vi "rotate phase angle of graph.vi"() -> ()   [LabVIEW 2012]
doc: "Rotates the phase of XY data from a Lockin Amplifier.\nWill average multiple input files.\nOnly use multiple files with the same scan parameters."
uses:
  <vilib>/Analysis/baseanly.llb/Mean (DBL).vi
  <vilib>/Utility/file.llb/Write To Spreadsheet File (DBL).vi
  <vilib>/Analysis/NI_AALBase.lvlib
panel:
  in  "Theta":dbl(knob) scale=0.0..360.0
  out "StdDev of Y":sgl
  out "#pages":i32
  out "#columns":i32
  out "#rows":i32
  in  "Put each data file you want to \naverage into a separate array element":string[](array[string])
  in  "Read in from array":bool
  out "array of new data":dbl[][](array[numeric])
  in  "Output to .xls file":bool
  in  "stop":bool
  out "Rotated Graph":T1(graph) caption="cpsgraph"
  in  "Original Graph":T2(graph) caption="cpsgraph"
  # "(pops up dialog box for name)"
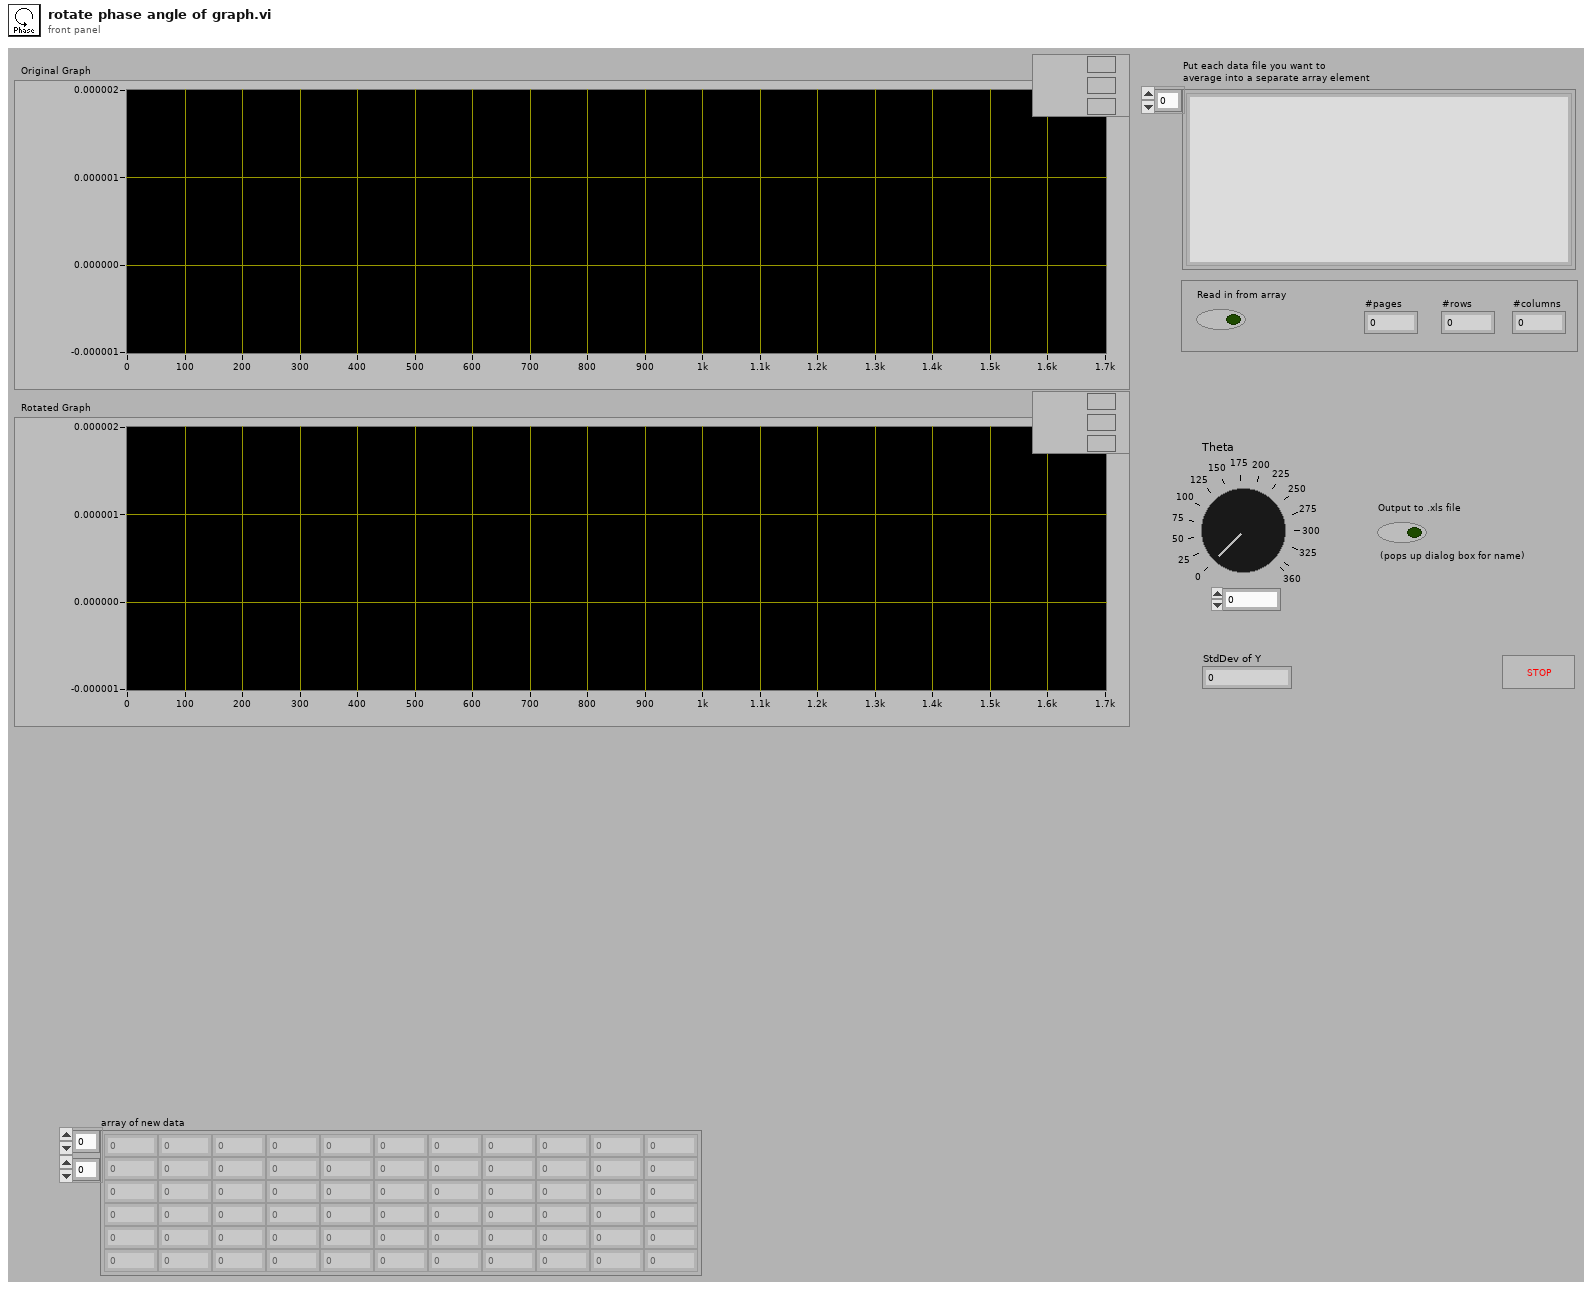
[diagram p1: front panel]
types:
  T1 = cluster{"point array":cluster{"x":dbl, "y":dbl}[]}[]
  T2 = typedef "Scan Driver.lvclass/Scan Graph.ctl" = cluster{"point array":cluster{"x":dbl, "y":dbl}[]}[]
  T3 = cluster{"point array":cluster{"x":dbl, "y":dbl}[]}
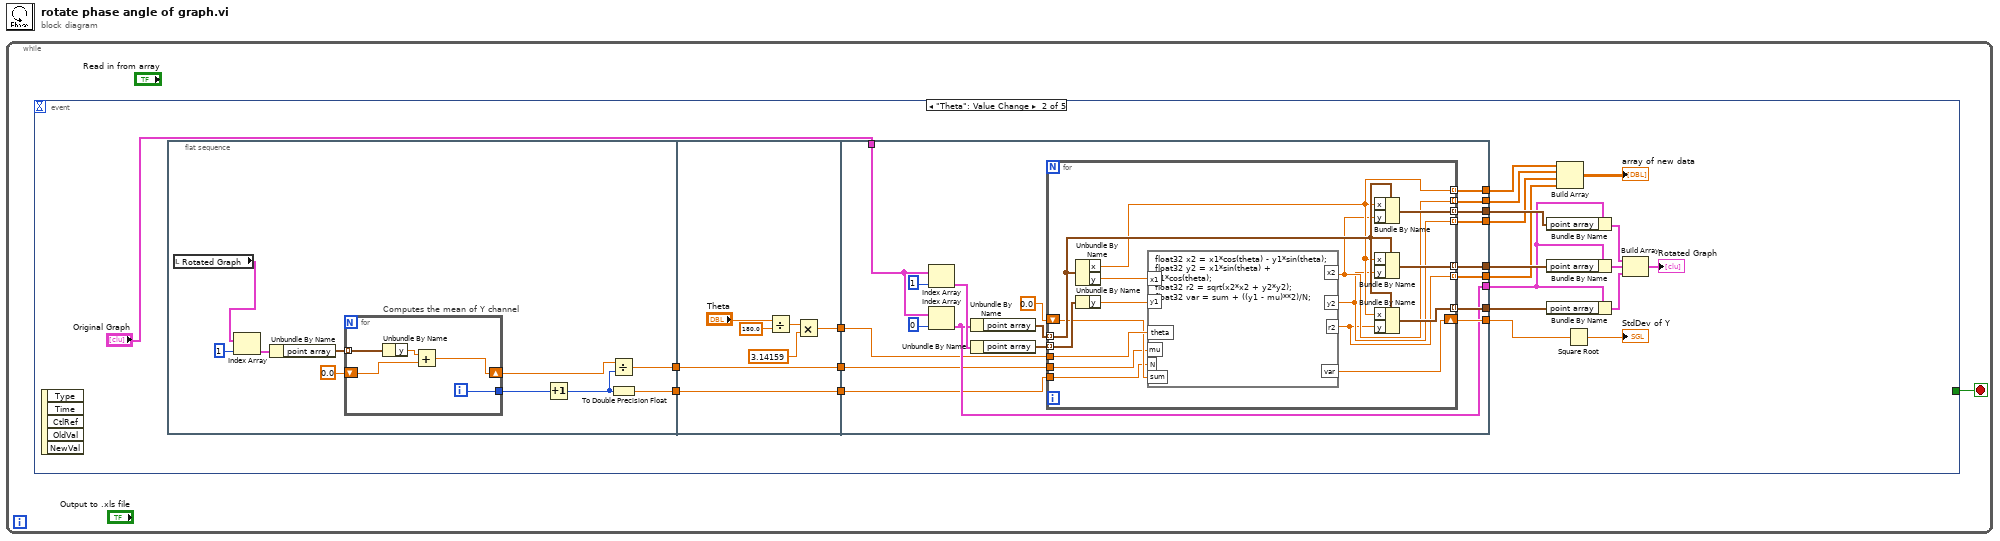
[diagram p0: block diagram]
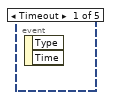
[diagram p2: hidden frame]
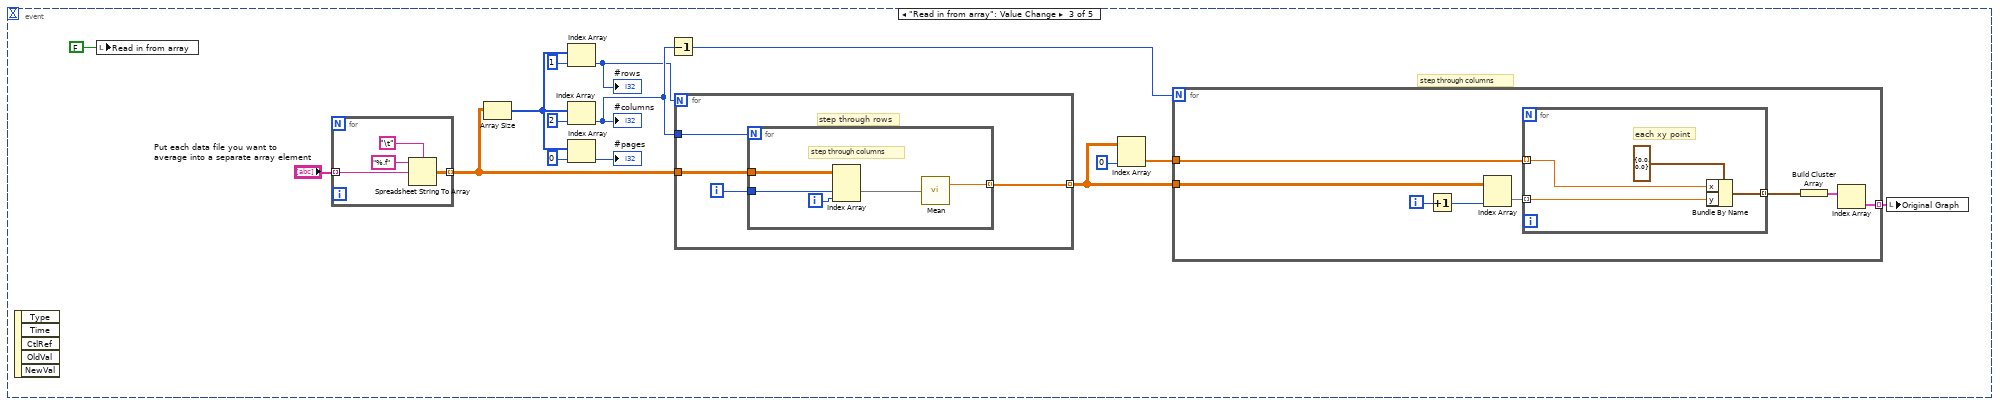
[diagram p3: hidden frame]
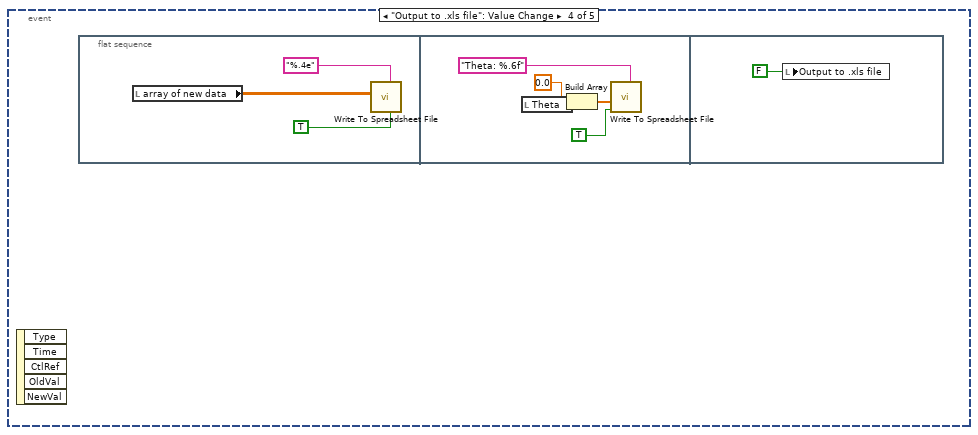
[diagram p4: hidden frame]
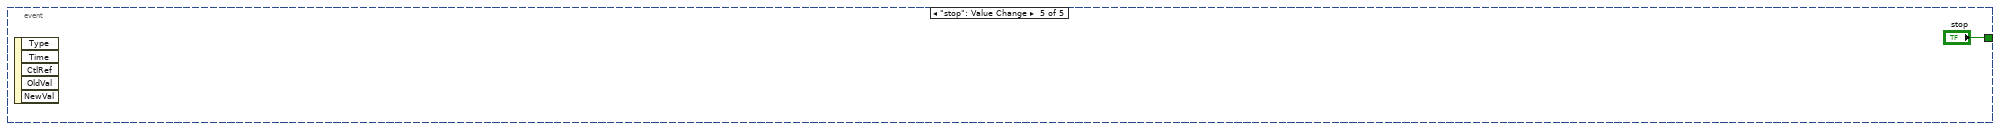
[diagram p5: hidden frame]
diagram:
  n1 = while {
    stop <- w1 stop-if-true
    n2 = event shown="[1] \"Theta\": Value Change" {
      selector: _ -> [_ _ _ _ _]
      dyn-events: _ -> [_ _ _ _ _]
      timeout: _ -> [_ _ _ _ _]
      tunnel: [_ _ _ _ "stop"] -> w1
      event Timeout {
        n3 = event-data() -> ()  [unwired: 1 in, 2 out]
      }
      event "Theta": Value Change {
        n4 = event-data() -> ()  [unwired: 1 in, 5 out]
        n5 = flat-sequence {
          tunnel: [w25] -> w6
          tunnel: [w24] -> w4
          tunnel: w6 -> [w39]
          tunnel: [w40] -> w5
          tunnel: w4 -> [w40]
          tunnel: [w39] -> w3
          tunnel: [w38] -> w2
          tunnel: [w63] -> w18
          tunnel: [w62] -> w17
          tunnel: [w61] -> w16
          tunnel: [w60] -> w15
          tunnel: [w59] -> w14
          tunnel: [w58] -> w13
          tunnel: [w57] -> w12
          tunnel: [w56] -> w10
          tunnel: "Original Graph" -> [w50]
          tunnel: [w49] -> w8
          tunnel: w5 -> [w48]
          tunnel: w3 -> [w47]
          tunnel: w2 -> [w46]
          frame #0 {
            n6 = local read "Rotated Graph"() -> (w23:T1)
            n7 = Index Array(array=w23, index=1) -> (element=w26:T3)
            n8 = Unbundle By Name(w26) -> ("point array"=w27:cluster{"x":dbl, "y":dbl}[])
            n9 = for "Computes the mean of Y channel" {
              tunnel: w27 -> [w34] mode=indexing
              shift-right: [w36] -> w30
              shift-left: 0.0 -> [w37]
              tunnel: [w35] -> w29
              i -> [w35]
              n10 = Unbundle By Name(w34) -> ("y"=w33:dbl)
              n11 = Add(x=w33, y=w37) -> (x+y=w36:dbl)
            }
            n12 = Increment(x=w29) -> (x+1=w31:i32)
            n13 = Divide(x=w30, y=w31) -> (x/y=w25:dbl)
            n14 = To Double Precision Float(number=w31) -> (double precision float=w24:dbl)
          }
          frame #1 {
            n15 = Divide(x="Theta", y=180.0) -> (x/y=w42:dbl)
            n16 = Multiply(x=w42, y=3.14159) -> (x*y=w38:dbl)
          }
          frame #2 {
            n17 = Index Array(array=w50, index=1) -> (element=w53:T3)
            n18 = Index Array(array=w50, index=0) -> (element=w49:T3)
            n19 = Unbundle By Name(w49) -> ("point array"=w52:cluster{"x":dbl, "y":dbl}[])
            n20 = Unbundle By Name(w53) -> ("point array"=w51:cluster{"x":dbl, "y":dbl}[])
            n21 = for {
              tunnel: w52 -> [w78] mode=indexing
              tunnel: w51 -> [w79] mode=indexing
              tunnel: w46 -> [w71]
              tunnel: [w77] -> w61 mode=indexing
              tunnel: [w76] -> w62 mode=indexing
              tunnel: [w75] -> w63 mode=indexing
              tunnel: [w74] -> w60 mode=indexing
              tunnel: [w70] -> w59 mode=indexing
              tunnel: [w69] -> w58 mode=indexing
              tunnel: [w68] -> w57 mode=indexing
              shift-right: [w67] -> w56
              shift-left: sgl 0.0 -> [w66]
              tunnel: w48 -> [w65]
              tunnel: w47 -> [w64]
              n22 = Unbundle By Name(w78) -> ("x"=w74:dbl, "y"=w73:dbl)
              n23 = Unbundle By Name(w79) -> ("y"=w72:dbl)
              n24 = formula code="float32 x2 = x1*cos(theta) - y1*sin(theta);\nfloat32 y2 = x1*sin(theta) + y1*cos(theta);\nfloat32 r2 = sqrt(x2*x2 + y2*y2);\nfloat32 var = sum + ((y1 - mu)**2)/N;"("x1"=w73, "y1"=w72, "theta"=w71, "mu"=w64, "N"=w65, "sum"=w66) -> ("x2"=w70:sgl, "y2"=w69:sgl, "r2"=w68:sgl, "var"=w67:sgl)
              n25 = Bundle By Name(cluster=w78, "x"=w74, "y"=w70) -> (w77:cluster{"x":dbl, "y":dbl})
              n26 = Bundle By Name(cluster=w78, "x"=w74, "y"=w69) -> (w76:cluster{"x":dbl, "y":dbl})
              n27 = Bundle By Name(cluster=w78, "x"=w74, "y"=w68) -> (w75:cluster{"x":dbl, "y":dbl})
            }
          }
        }
        n28 = Bundle By Name(cluster=w8, "point array"=w16) -> (w19:T3)
        n29 = Bundle By Name(cluster=w8, "point array"=w17) -> (w20:T3)
        n30 = Bundle By Name(cluster=w8, "point array"=w18) -> (w21:T3)
        n31 = Build Array(w15, w14, w13, w12) -> (→"array of new data":dbl[][])
        n32 = Square Root(x=w10) -> (sqrt(x)=→"StdDev of Y":sgl)
        n33 = Build Array(w19, w20, w21) -> (→"Rotated Graph":T1)
      }
      event "Read in from array": Value Change {
        # "step through columns"
        n34 = event-data() -> ()  [unwired: 1 in, 5 out]
        n35 = local write "Read in from array"(FALSE ("Read in from array")) -> ()
        n36 = for {
          tunnel: "Put each data file you want to \naverage into a separate array element" -> [w119] mode=indexing
          tunnel: [w118] -> w81 mode=indexing
          n37 = Spreadsheet String To Array(delimiter (Tab)="\t", format string="%.f", spreadsheet string=w119) -> (array=w118:dbl[][])  [unwired: 1 in]
        }
        n38 = Array Size(array=w81) -> (size(s)=w91:i32[])
        n39 = Index Array(array=w91, index=1) -> (element=w80:i32)
        "#rows" <- w80
        n40 = Index Array(array=w91, index=2) -> (element=w87:i32)
        "#columns" <- w87
        n41 = Index Array(array=w91, index=0) -> (element=→"#pages":i32)
        n42 = Decrement(x=w87) -> (x-1=w86:i32)
        n43 = for {
          N: w80 -> [_]
          tunnel: w81 -> [w110]
          tunnel: [w109] -> w83 mode=indexing
          tunnel: w87 -> [w108]
          i -> [w107]
          # "step through rows"
          n44 = for {
            N: w108 -> [_]
            tunnel: w110 -> [w114]
            tunnel: [w115] -> w109 mode=indexing
            tunnel: w107 -> [w113]
            i -> [w112]
            # "step through columns"
            n45 = Index Array(array=w114, index (dim 1)=w113, index (dim 2)=w112) -> (element=w111:dbl[])  [unwired: 1 in]
            n46 = call-poly <vilib>:"Mean.vi"("X"=w111) -> ("mean"=w115:dbl)  [unwired: 1 out]
          }
        }
        n47 = Index Array(array=w83, index (col)=0 ("disabled index (col)")) -> (element=w82:dbl[])  [unwired: 1 in]
        n48 = for {
          N: w86 -> [_]
          tunnel: w83 -> [w99]
          tunnel: [w95] -> w85 mode=indexing
          tunnel: w82 -> [w98]
          i -> [w100]
          n49 = Increment(x=w100) -> (x+1=w102:i32)
          n50 = Index Array(array=w99, index (col)=w102) -> (element=w101:dbl[])  [unwired: 1 in]
          n51 = for {
            tunnel: w98 -> [w106] mode=indexing
            tunnel: w101 -> [w105] mode=indexing
            tunnel: [w104] -> w97 mode=indexing
            # "each xy point"
            n52 = Bundle By Name(cluster=cluster{"x":dbl, "y":dbl} {"x"=0.0, "y"=0.0} ("element"), "x"=w106, "y"=w105) -> (w104:cluster{"x":dbl, "y":dbl})
          }
          n53 = Build Cluster Array(w97) -> (w96:cluster{cluster{"x":dbl, "y":dbl}[]}[])
          n54 = Index Array(array=w96) -> (element=w95:cluster{cluster{"x":dbl, "y":dbl}[]})  [unwired: 1 in]
        }
        n55 = local write "Original Graph"(w85) -> ()
      }
      event "Output to .xls file": Value Change {
        n56 = event-data() -> ()  [unwired: 1 in, 5 out]
        n57 = flat-sequence {
          frame #0 {
            n58 = local read "array of new data"() -> (w122:dbl[][])
            n59 = call-poly <vilib>:"Write To Spreadsheet File.vi"("transpose? (no:F)"=TRUE, "format (%.3f)"="%.4e", "2D data"=w122) -> ()  [unwired: 5 in, 1 out]
          }
          frame #1 {
            n60 = local read "Theta"() -> (w126:dbl)
            n61 = Build Array(0.0, w126) -> (w123:dbl[])
            n62 = call-poly <vilib>:"Write To Spreadsheet File.vi"("format (%.3f)"="Theta: %.6f", "append to file? (new file:F)"=TRUE, "1D data"=w123) -> ()  [unwired: 5 in, 1 out]
          }
          frame #2 {
            n63 = local write "Output to .xls file"(FALSE ("Output to file")) -> ()
          }
        }
      }
      event "stop": Value Change {
        n64 = event-data() -> ()  [unwired: 1 in, 5 out]
      }
    }
  }
